vi "Next Submission.vi"(8 "error in (no error)":errorcluster) -> (0 "error out":errorcluster, 3 "submission":i32, 5 "Profile URL":string)   [LabVIEW 2024, in "Wordle Scorer.lvlib"]
uses:
  Wordle Scorer.lvlib
  Next Submission.ctl
  Error Response.ctl
  Next Scoring Request.ctl
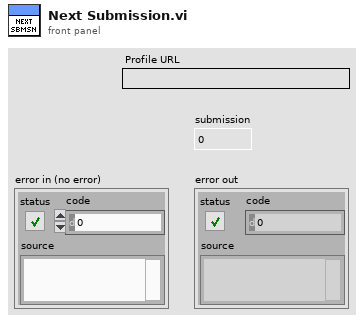
[diagram p1: front panel]
types:
  T1 = typedef "Wordle Scorer.lvlib/Next Scoring Request.ctl" = cluster{"scorer":string, "key":string, "challenges":i32[]}
  T2 = typedef "Wordle Scorer.lvlib/Next Submission.ctl" = cluster{"code":i32, "submission":i32}
  T3 = typedef "Wordle Scorer.lvlib/Error Response.ctl" = cluster{"code":i32, "message":string}
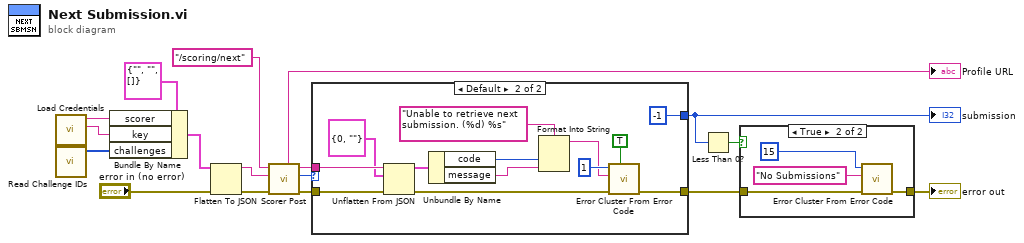
[diagram p0: block diagram]
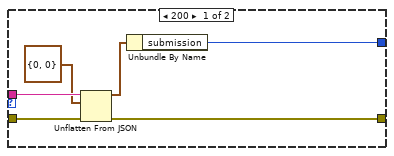
[diagram p2: hidden frame]
diagram:
  n1 = call "Load Credentials.vi"() -> ("Key"=w9:string, "ID"=w11:string)  [unwired: 9 in, 1 out]
  n2 = call "Read Challenge IDs.vi"() -> ("IDs"=w10:i32[])  [unwired: 10 in, 1 out]
  n3 = Bundle By Name(cluster=T1 {"scorer"="", "key"="", "challenges"=[]} ("Next Scoring Request"), "scorer"=w11, "key"=w9, "challenges"=w10) -> (w8:T1)
  n4 = Flatten To JSON(anything=w8, error in (no error)="error in (no error)") -> (JSON string=w7:string, 11:w5:errorcluster)  [unwired: 1 in]
  n5 = call "Scorer Post.vi"("error in (no error)"=w5, "buffer"=w7, "Path"="/scoring/next") -> ("error out"=w16:errorcluster, "Status"=w15:i32, "Content"=w14:string, "Profile URL"=→"Profile URL":string)  [unwired: 5 in]
  n6 = case shown="Default" w15 {
    tunnel: w16 -> [w20 w34]
    tunnel: w14 -> [w23 w36]
    tunnel: [w18 w30] -> w2
    tunnel: [w19 -1 ("submission")] -> w3
    frame 200 {
      n7 = Unflatten From JSON(JSON string=w23, type and defaults=T2 {"code"=0, "submission"=0} ("Next Submission"), error in (no error)=w20) -> (value=w21:T2, error out=w18:errorcluster)  [unwired: 4 in]
      n8 = Unbundle By Name(w21) -> ("submission"=w19:i32)
    }
    frame Default {
      n9 = Unflatten From JSON(JSON string=w36, type and defaults=T3 {"code"=0, "message"=""} ("Error Response"), error in (no error)=w34) -> (value=w35:T3, error out=w31:errorcluster)  [unwired: 4 in]
      n10 = Unbundle By Name(w35) -> ("code"=w25:i32, "message"=w24:string)
      n11 = Format Into String(format string="Unable to retrieve next submission. (%d) %s", w25, w24) -> (resulting string=w27:string)  [unwired: 2 in, 1 out]
      n12 = call <vilib>:"Error Cluster From Error Code.vi"("show call chain? (False)"=TRUE, "error in (no error)"=w31, "error message (\"\")"=w27, "error code (0)"=1) -> ("error out"=w30:errorcluster)  [unwired: 5 in]
    }
  }
  "submission" <- w3
  n13 = Less Than 0?(x=w3) -> (x < 0?=w4:bool)
  n14 = case shown="True" w4 {
    tunnel: w2 -> [w37 w41]
    tunnel: [w37 w40] -> w1
    frame False {
    }
    frame True {
      n15 = call <vilib>:"Error Cluster From Error Code.vi"("error in (no error)"=w41, "error message (\"\")"="No Submissions" ("error message (\"\")"), "error code (0)"=15) -> ("error out"=w40:errorcluster)  [unwired: 6 in]
    }
  }
  "error out" <- w1
